vi "Best y.vi"(9 "Maior intervalo":bool, 10 "IA State":T2) -> (0 "pilha output (merged)":T1[](array[typedef]), 1 "Vetor de segmentos ordenado":T1[](array[typedef]), 2 "Vetor de segmentos (sombras)":T1[](array[typedef]), 3 "Vetor de gaps":T1[](array[typedef]), 4 "Best y":dbl, 5 "Eclipse":bool)   [LabVIEW 2016]
uses:
  Core/AI Input.ctl
  Core/AI Robot.ctl
  Intel/Functions Enum.ctl
  Core/AI Ball.ctl
  Core/Field Size.ctl
  Core/AI Judge.ctl
  Intel/Command Enum.ctl
  segment.ctl
panel:
  in  "inimigos":bool=TRUE
  in  "eclipse angle eps":dbl=0.035 format="%#_13g"
  # "Maior ângulo"
  # "amigos"
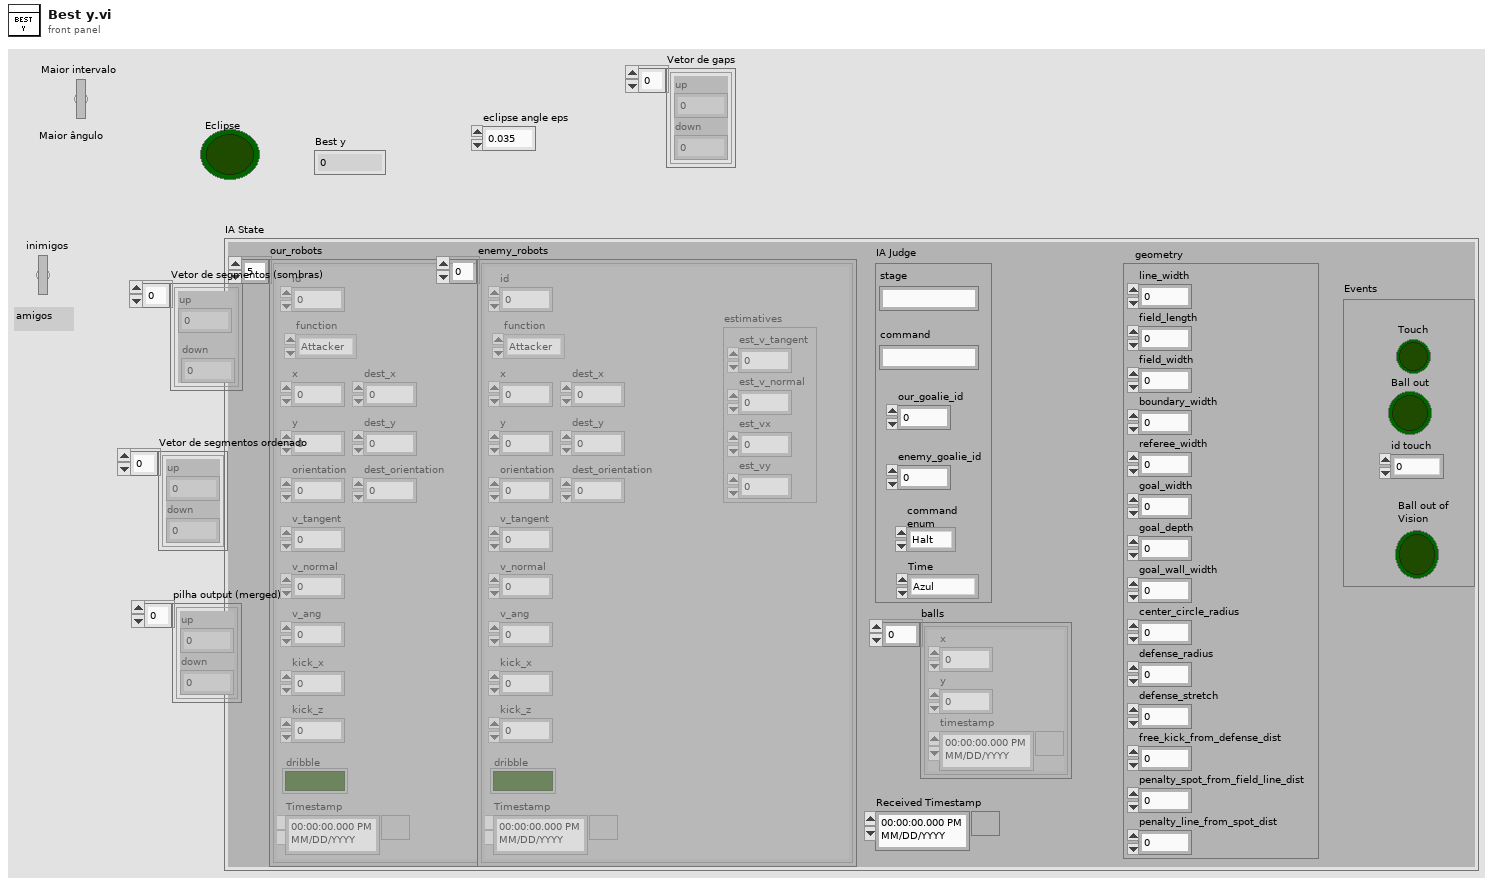
[diagram p1: front panel]
types:
  T1 = typedef "segment.ctl" = cluster{"up":dbl, "down":dbl}
  T2 = typedef "AI Input.ctl" = cluster{"our_robots":T3[], "enemy_robots":T3[], "balls":T5[], "geometry":T6, "IA Judge":T7, "Received Timestamp":timestamp, "Events":cluster{"Touch":bool, "Ball out":bool, "id touch":dbl, "Ball out of \nVision":bool}}
  T3 = typedef "AI Robot.ctl" = cluster{"id":u32, "function":T4, "x":dbl, "y":dbl, "orientation":dbl, "v_tangent":dbl, "v_normal":dbl, "v_ang":dbl, "kick_x":dbl, "kick_z":dbl, "dribble":bool, "Timestamp":timestamp, "dest_x":dbl, "dest_y":dbl, "dest_orientation":dbl, "estimatives":cluster{"est_v_tangent":dbl, "est_v_normal":dbl, "est_vx":dbl, "est_vy":dbl}}
  T4 = typedef "Functions Enum.ctl" = enum16{"Attacker", "Goalie", "Defender", "Striker", "Goto 0", "Dummy", "ZigZag"}
  T5 = typedef "AI Ball.ctl" = cluster{"x":dbl, "y":dbl, "timestamp":timestamp}
  T6 = typedef "Field Size.ctl" = cluster{"line_width":u32, "field_length":u32, "field_width":u32, "boundary_width":u32, "referee_width":u32, "goal_width":u32, "goal_depth":u32, "goal_wall_width":u32, "center_circle_radius":u32, "defense_radius":u32, "defense_stretch":u32, "free_kick_from_defense_dist":u32, "penalty_spot_from_field_line_dist":u32, "penalty_line_from_spot_dist":u32}
  T7 = typedef "AI Judge.ctl" = cluster{"stage":string, "command":string, "our_goalie_id":dbl, "enemy_goalie_id":dbl, "command\nenum":T8, "Time":enum16{"Azul", "Amarelo"}}
  T8 = typedef "Command Enum.ctl" = enum16{"Halt", "Stop", "Force Start", "PKA Normal Start", "Prepare Kickoff Ally", "PKE Normal Start", "Prepare Kickoff Enemy", "Prepare Penalty Ally", "PPA Normal Start", "Prepare Penalty Enemy", "PPE Normal Start", "Direct Free Enemy", "Direct Free Ally", "Indirect Free Enemy", "Indirect Free Ally", "Timeout Enemy", "Timeout Ally", "Goal Enemy", "Goal Ally", "Ball Placement Enemy", "Ball Placement Ally", "None"}
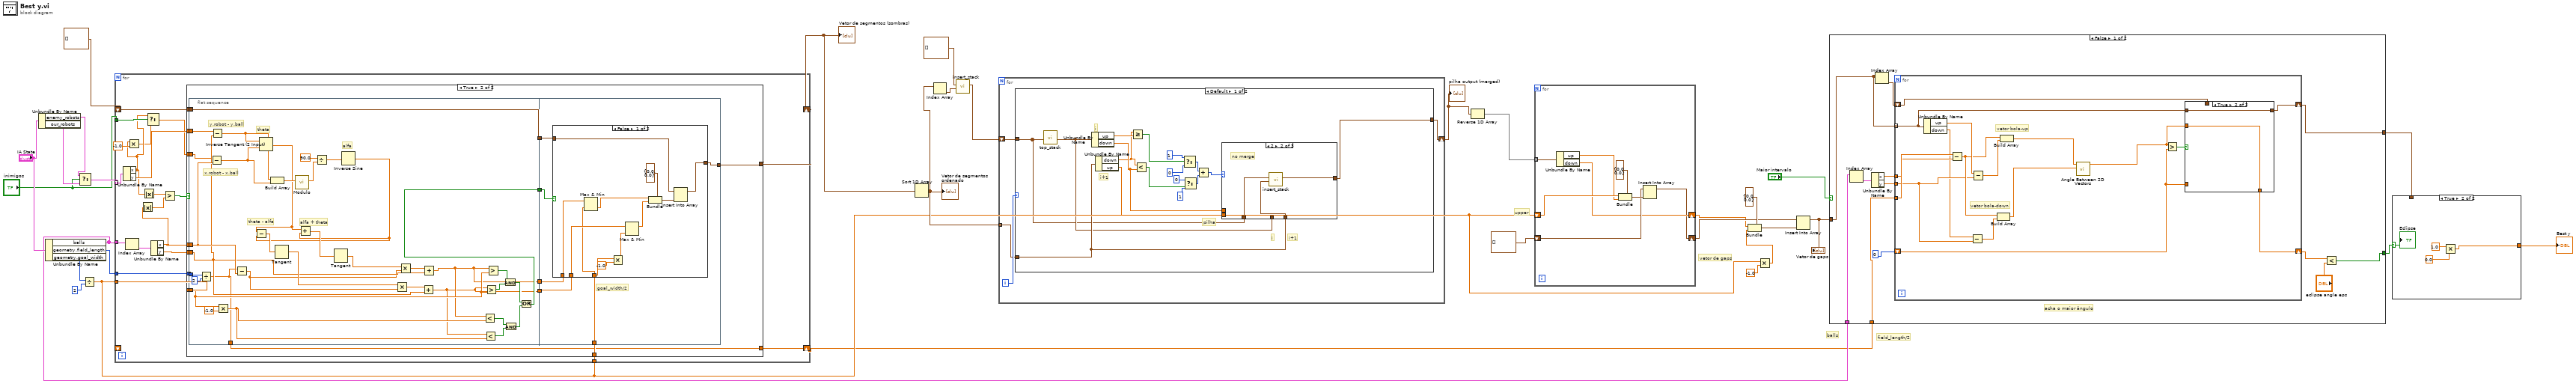
[diagram p0: block diagram]
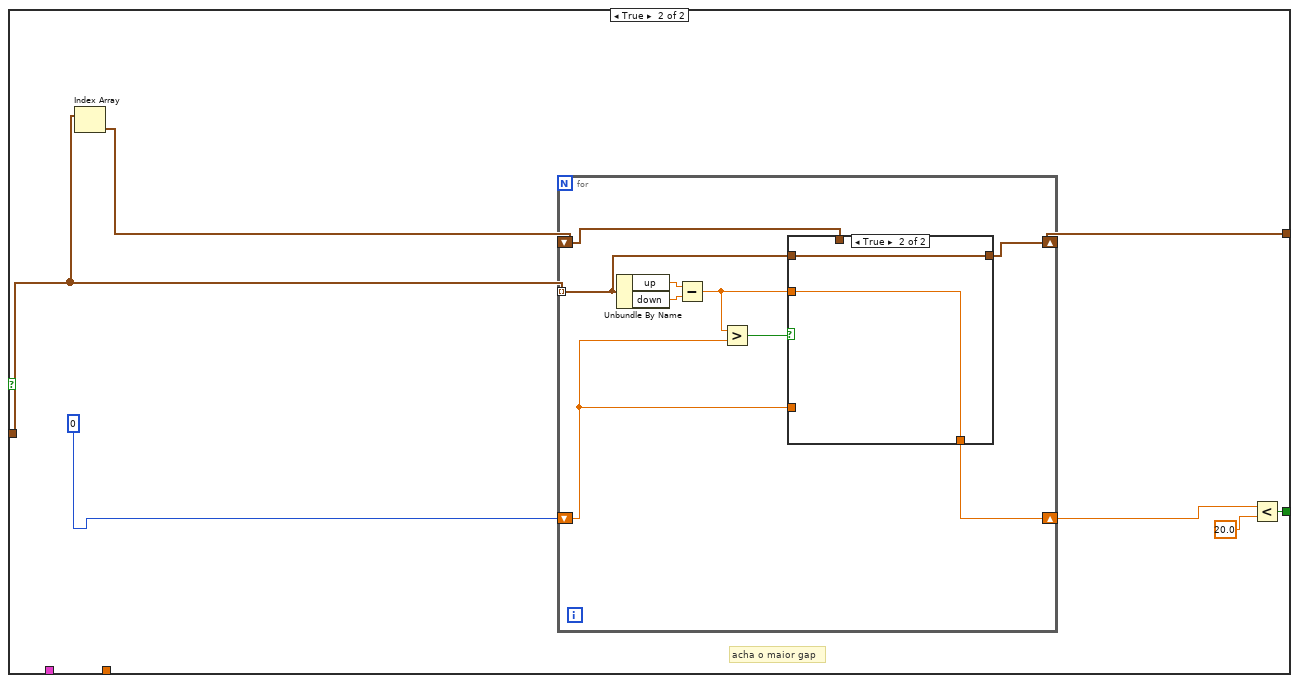
[diagram p3: hidden frame]
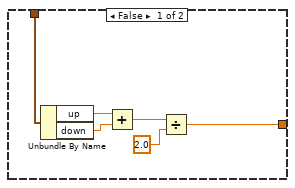
[diagram p5: hidden frame]
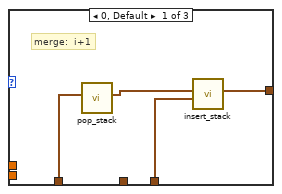
[diagram p6: hidden frame]
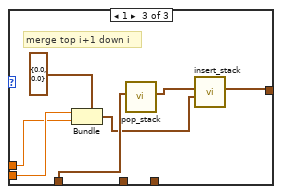
[diagram p7: hidden frame]
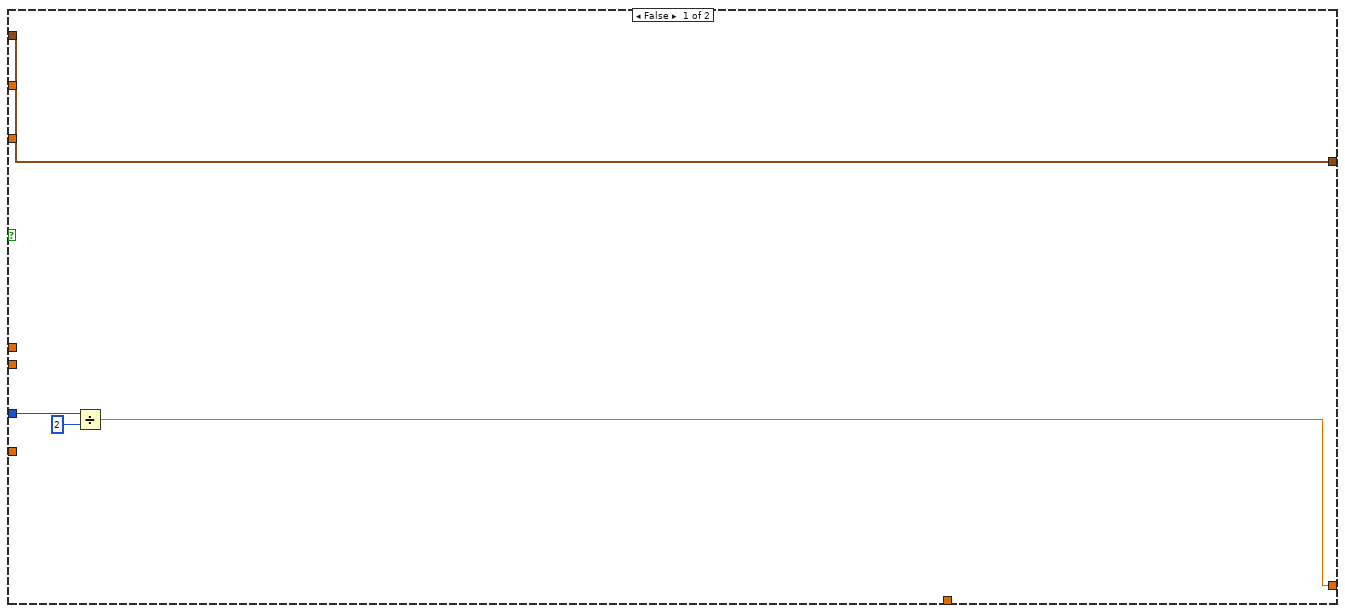
[diagram p9: hidden frame]
diagram:
  # "field_length/2"
  # "balls"
  # "vetor de gaps"
  # "upper"
  n1 = Unbundle By Name("IA State") -> ("enemy_robots"=w4:T3[], "our_robots"=w3:T3[])
  n2 = Unbundle By Name("IA State") -> ("balls"=w7:T5[], "geometry.field_length"=w30:u32, "geometry.goal_width"=w27:u32)
  n3 = Select(t=w4, s="inimigos", f=w3) -> (s? t:f=w2:T3[])
  n4 = Divide(x=w27, y=u32 2 ("x")) -> (x/y=w13:dbl)
  n5 = for {
    tunnel: w7 -> [w50]
    shift-right: [w47] -> w12
    shift-left: T1[] [] -> [w46]
    tunnel: w30 -> [w45]
    tunnel: w13 -> [w44]
    tunnel: w13 -> [w40]
    shift-right: [w39] -> w5
    shift-left: _ -> [_]
    tunnel: w2 -> [w38] mode=indexing
    tunnel: "inimigos" -> [w35]
    n6 = Unbundle By Name(w38) -> ("x"=w34:dbl, "y"=w37:dbl)
    n7 = Index Array(array=w50) -> (element=w51:T5)  [unwired: 1 in]
    n8 = Multiply(x=w34, y=-1.0) -> (x*y=w33:dbl)
    n9 = Absolute Value(x=w34) -> (abs(x)=w41:dbl)
    n10 = Select(t=w34, s=w35, f=w33) -> (s? t:f=w32:dbl)
    n11 = Unbundle By Name(w51) -> ("x"=w43:dbl, "y"=w48:dbl)
    n12 = Absolute Value(x=w43) -> (abs(x)=w42:dbl)
    n13 = Greater?(x=w41, y=w42) -> (0:w49:bool)
    n14 = case shown="True" w49 {
      tunnel: w48 -> [_ w69]
      tunnel: w43 -> [_ w67]
      tunnel: [w55 w60] -> w47
      tunnel: w46 -> [w55 w62]
      tunnel: w45 -> [w54 w68]
      tunnel: w44 -> [_ w66]
      tunnel: w40 -> [_ w59]
      tunnel: [w52 w58] -> w39
      tunnel: w37 -> [_ w57]
      tunnel: w32 -> [_ w56]
      frame False {
        n15 = Divide(x=w54, y=u32 2) -> (x/y=w52:dbl)
      }
      frame True {
        n16 = flat-sequence {
          tunnel: w57 -> [w104]
          tunnel: w69 -> [w75]
          tunnel: w68 -> [w100]
          tunnel: w67 -> [w98]
          tunnel: w66 -> [w84]
          tunnel: [w73] -> w65
          tunnel: [w72] -> w64
          tunnel: [w85] -> w63
          tunnel: w62 -> [w78]
          tunnel: [w78] -> w61
          tunnel: [w71] -> w58
          tunnel: w56 -> [w70]
          tunnel: w65 -> [w108]
          tunnel: w64 -> [w107]
          tunnel: w63 -> [w109]
          tunnel: w61 -> [w110]
          tunnel: [w106] -> w60
          tunnel: w59 -> [w105]
          frame #0 {
            # "theta - alfa"
            # "alfa + theta"
            # "theta"
            # "alfa"
            # "x.robot - x.ball"
            # "y.robot - y.ball"
            n17 = Divide(x=w100, y=u32 2 ("x")) -> (x/y=w71:dbl)
            n18 = Subtract(x=w70, y=w98) -> (x-y=w82:dbl)
            n19 = Subtract(x=w104, y=w75) -> (x-y=w83:dbl)
            n20 = Multiply(x=w84, y=-1.0) -> (x*y=w90:dbl)
            n21 = Subtract(x=w71, y=w98) -> (x-y=w74:dbl)
            n22 = Inverse Tangent (2 Input)(1:w82, 2:w83) -> (0:w81:dbl)
            n23 = Build Array(w83, w82) -> (w103:dbl[])
            n24 = call "Modulo.vi"("2D vector"=w103) -> ("Modulo"=w101:dbl)  [unwired: 10 in]
            n25 = Divide(x=90.0, y=w101) -> (x/y=w80:dbl)
            n26 = Inverse Sine(1:w80) -> (0:w79:dbl)
            n27 = Subtract(x=w81, y=w79) -> (x-y=w95:dbl)
            n28 = Tangent(1:w95) -> (0:w94:dbl)
            n29 = Add(x=w81, y=w79) -> (x+y=w97:dbl)
            n30 = Tangent(1:w97) -> (0:w96:dbl)
            n31 = Multiply(x=w94, y=w74) -> (x*y=w76:dbl)
            n32 = Multiply(x=w96, y=w74) -> (x*y=w77:dbl)
            n33 = Add(x=w76, y=w75) -> (x+y=w72:dbl)
            n34 = Add(x=w77, y=w75) -> (x+y=w73:dbl)
            n35 = Less?(x=w73, y=w90) -> (x < y?=w89:bool)
            n36 = Less?(x=w72, y=w90) -> (x < y?=w88:bool)
            n37 = Greater?(x=w72, y=w84) -> (0:w92:bool)
            n38 = Greater?(x=w73, y=w84) -> (0:w93:bool)
            n39 = And(x=w93, y=w92) -> (x .and. y?=w87:bool)
            n40 = And(x=w89, y=w88) -> (x .and. y?=w86:bool)
            n41 = Or(x=w87, y=w86) -> (x .or. y?=w85:bool)
          }
          frame #1 {
            # "goal_width/2"
            n42 = case shown="False" w109 {
              tunnel: [w119 w122] -> w106
              tunnel: w110 -> [w118 w122]
              tunnel: w108 -> [w117 _]
              tunnel: w107 -> [w115 _]
              tunnel: w105 -> [w114 _]
              frame False {
                n43 = Max & Min(x=w117, y=w114) -> (min(x,y)=w116:dbl)  [unwired: 1 out]
                n44 = Multiply(x=w114, y=-1.0) -> (x*y=w112:dbl)
                n45 = Max & Min(x=w115, y=w112) -> (max(x,y)=w111:dbl)  [unwired: 1 out]
                n46 = Bundle(cluster=T1 {"up"=0.0, "down"=0.0} ("segment 2"), "up"=w116, "down"=w111) -> (w120:T1)
                n47 = Insert Into Array(array=w118, new element=w120) -> (w119:T1[])  [unwired: 1 in]
              }
              frame True {
              }
            }
          }
        }
      }
    }
  }
  "Vetor de segmentos (sombras)" <- w12
  n48 = Sort 1D Array(array=w12) -> (sorted array=w26:T1[])
  "Vetor de segmentos ordenado" <- w26
  n49 = Index Array(array=w26) -> (element=w25:T1)  [unwired: 1 in]
  n50 = call "insert_stack.vi"("novo elemento"=w25, "pilha input"=T1[] []) -> ("pilha output"=w23:T1[])  [unwired: 9 in]
  n51 = for {
    shift-right: [w123] -> w22
    shift-left: w23 -> [w125]
    tunnel: w26 -> [w124] mode=indexing
    i -> [w126]
    n52 = case shown="Default" w126 {
      tunnel: w125 -> [w130 w158]
      tunnel: w124 -> [w133 _]
      tunnel: [w131 w158] -> w123
      frame Default {
        # "pilha"
        # "i+1"
        # "i"
        # "i+1"
        # "i"
        n53 = call "top_stack.vi"("pilha input"=w130) -> ("top"=w132:T1)  [unwired: 10 in]
        n54 = Unbundle By Name(w132) -> ("up"=w129:dbl, "down"=w134:dbl)
        n55 = Unbundle By Name(w133) -> ("down"=w128:dbl, "up"=w135:dbl)
        n56 = Greater Or Equal?(x=w128, y=w129) -> (x >= y?=w127:bool)
        n57 = Less?(x=w128, y=w134) -> (x < y?=w137:bool)
        n58 = Select(t=1, s=w127, f=0) -> (s? t:f=w139:i32)
        n59 = Select(t=0, s=w137, f=1) -> (s? t:f=w138:i32)
        n60 = Add(x=w139, y=w138) -> (x+y=w136:i32)
        n61 = case shown="2" w136 {
          tunnel: w135 -> [_ _ w156]
          tunnel: w134 -> [_ _ w155]
          tunnel: w132 -> [_ _ _]
          tunnel: w133 -> [w144 w149 _]
          tunnel: [w147 w148 w151] -> w131
          tunnel: w130 -> [w146 w150 w154]
          frame 0, Default {
            # "merge:  i+1"
            n62 = call "pop_stack.vi"("pilha input"=w146) -> ("pilha output"=w145:T1[])  [unwired: 9 in]
            n63 = call "insert_stack.vi"("novo elemento"=w144, "pilha input"=w145) -> ("pilha output"=w147:T1[])  [unwired: 9 in]
          }
          frame 2 {
            # "no merge"
            n64 = call "insert_stack.vi"("novo elemento"=w149, "pilha input"=w150) -> ("pilha output"=w148:T1[])  [unwired: 9 in]
          }
          frame 1 {
            # "merge top i+1 down i"
            n65 = Bundle(cluster=T1 {"up"=0.0, "down"=0.0} ("segment 2"), "up"=w156, "down"=w155) -> (w152:T1)
            n66 = call "pop_stack.vi"("pilha input"=w154) -> ("pilha output"=w153:T1[])  [unwired: 9 in]
            n67 = call "insert_stack.vi"("novo elemento"=w152, "pilha input"=w153) -> ("pilha output"=w151:T1[])  [unwired: 9 in]
          }
        }
      }
      frame 0 {
      }
    }
  }
  "pilha output (merged)" <- w22
  n68 = Reverse 1D Array(array=w22) -> (reversed array=w21:T1[])
  n69 = for {
    tunnel: w21 -> [w166] mode=indexing
    shift-right: [w160] -> w17
    shift-left: T1[] [] -> [w162]
    shift-right: [w161] -> w16
    shift-left: w13 -> [w163]
    n70 = Unbundle By Name(w166) -> ("up"=w159:dbl, "down"=w161:dbl)
    n71 = Bundle(cluster=T1 {"up"=0.0, "down"=0.0} ("segment 2"), "up"=w163, "down"=w159) -> (w165:T1)
    n72 = Insert Into Array(array=w162, new element=w165) -> (w160:T1[])  [unwired: 1 in]
  }
  n73 = Multiply(x=w13, y=-1.0) -> (x*y=w14:dbl)
  n74 = Bundle(cluster=T1 {"up"=0.0, "down"=0.0} ("segment 2"), "up"=w16, "down"=w14) -> (w19:T1)
  n75 = Insert Into Array(array=w17, new element=w19) -> (w8:T1[])  [unwired: 1 in]
  "Vetor de gaps" <- w8
  n76 = case shown="False" "Maior intervalo" {
    tunnel: [w168 w203] -> w11
    tunnel: [w167 w201] -> w10
    tunnel: w8 -> [w176 w202]
    tunnel: w7 -> [w175 _]
    tunnel: w5 -> [w171 _]
    frame False {
      # "acha o maior ângulo"
      n77 = Index Array(array=w175) -> (element=w174:T5)  [unwired: 1 in]
      n78 = Unbundle By Name(w174) -> ("x"=w173:dbl, "y"=w172:dbl)
      n79 = Index Array(array=w176) -> (element=w177:T1)  [unwired: 1 in]
      n80 = for {
        tunnel: w176 -> [w193] mode=indexing
        shift-right: [w194] -> w170
        shift-left: 0 -> [w179]
        shift-right: [w192] -> w167
        shift-left: w177 -> [w191]
        tunnel: w173 -> [w189]
        tunnel: w172 -> [w185]
        tunnel: w171 -> [w190]
        # "vetor bola-down"
        # "vetor bola-up"
        n81 = Unbundle By Name(w193) -> ("up"=w188:dbl, "down"=w184:dbl)
        n82 = Subtract(x=w190, y=w189) -> (x-y=w186:dbl)
        n83 = Subtract(x=w184, y=w185) -> (x-y=w183:dbl)
        n84 = Subtract(x=w188, y=w185) -> (x-y=w187:dbl)
        n85 = Build Array(w186, w183) -> (w181:dbl[])
        n86 = Build Array(w186, w187) -> (w182:dbl[])
        n87 = call "Angle Between 2D Vectors.vi"("Array"=w181, "Array 2"=w182) -> ("Numeric"=w180:dbl)  [unwired: 9 in]
        n88 = Greater?(x=w180, y=w179) -> (0:w195:bool)
        n89 = case shown="True" w195 {
          tunnel: w180 -> [_ w199]
          tunnel: [w196 w199] -> w194
          tunnel: w193 -> [_ w198]
          tunnel: [w197 w198] -> w192
          tunnel: w191 -> [w197 _]
          tunnel: w179 -> [w196 _]
          frame False {
          }
          frame True {
          }
        }
      }
      n90 = Less?(x=w170, y="eclipse angle eps") -> (x < y?=w168:bool)
    }
    frame True {
      # "acha o maior gap"
      n91 = Index Array(array=w202) -> (element=w205:T1)  [unwired: 1 in]
      n92 = for {
        tunnel: w202 -> [w210] mode=indexing
        shift-right: [w211] -> w204
        shift-left: 0 -> [w208]
        shift-right: [w209] -> w201
        shift-left: w205 -> [w207]
        n93 = Unbundle By Name(w210) -> ("up"=w215:dbl, "down"=w214:dbl)
        n94 = Subtract(x=w215, y=w214) -> (x-y=w212:dbl)
        n95 = Greater?(x=w212, y=w208) -> (0:w213:bool)
        n96 = case shown="True" w213 {
          tunnel: w212 -> [_ w219]
          tunnel: [w217 w219] -> w211
          tunnel: w210 -> [_ w218]
          tunnel: [w216 w218] -> w209
          tunnel: w208 -> [w217 _]
          tunnel: w207 -> [w216 _]
          frame False {
          }
          frame True {
          }
        }
      }
      n97 = Less?(x=w204, y=20.0) -> (x < y?=w203:bool)
    }
  }
  n98 = case shown="True" w11 {
    selector: w11 -> [_ w229]
    tunnel: w10 -> [w221 _]
    tunnel: [w220 w226] -> w9
    frame False {
      n99 = Unbundle By Name(w221) -> ("up"=w222:dbl, "down"=w223:dbl)
      n100 = Add(x=w222, y=w223) -> (x+y=w224:dbl)
      n101 = Divide(x=w224, y=2.0) -> (x/y=w220:dbl)
    }
    frame True {
      n102 = Multiply(x=1.0, y=0.0) -> (x*y=w226:dbl)
      "Eclipse" <- w229
    }
  }
  "Best y" <- w9
